vi "CryptoNight-ParseLine.vi"(11 "line":string) -> (3 "Array":u32[](array[numeric]))   [LabVIEW 2017]
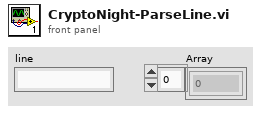
[diagram p1: front panel]
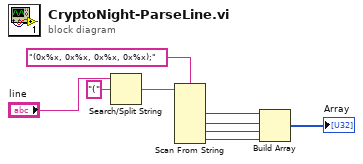
[diagram p0: block diagram]
diagram:
  n1 = Search/Split String(string="line", search string/char (-)="(") -> (match + rest of string=w8:string)  [unwired: 1 in, 2 out]
  n2 = Scan From String(format string="(0x%x, 0x%x, 0x%x, 0x%x);", input string=w8) -> (output 1=w1:u32, output 2=w2:u32, output 3=w3:u32, output 4=w4:u32)  [unwired: 6 in, 3 out]
  n3 = Build Array(w1, w2, w3, w4) -> (→"Array":u32[])
